vi "FTP_StatusBar.vi"(2 "i":i32, 3 "N":i32) -> (1 "Stop out":bool)   [LabVIEW 2012]
panel:
  in  "Stop":bool
  out "Progress":u8(slide) scale=0.0..100.0
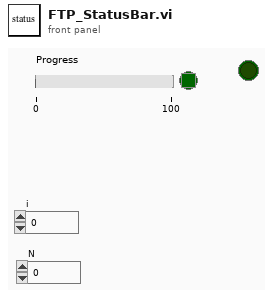
[diagram p1: front panel]
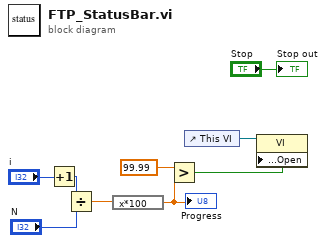
[diagram p0: block diagram]
diagram:
  n1 = Increment(x="i") -> (x+1=w8:i32)
  n2 = Divide(x=w8, y="N") -> (x/y=w6:dbl)
  n3 = expression code="x*100"(w6) -> (w4:dbl)
  "Progress" <- w4
  n4 = Greater?(x=99.99, y=w4) -> (0:w3:bool)
  n5 = control-ref of="This VI"() -> (w5:refnum<vi>)
  n6 = property class="VI"(reference=w5, "Front Panel.Open"=w3) -> ()  [unwired: 1 in, 2 out]
  "Stop out" <- "Stop"
